vi "Read Object List.vi"(8 "error in (no error)":errorcluster, 11 "file refnum":T1) -> (0 "error out":errorcluster, 2 "Mandatory Object List":u16[](array[numeric]), 3 "Optional Object List":u16[](array[numeric]))   [LabVIEW 2013]
uses:
  <vilib>/Utility/config.llb/Config Data RefNum.ctl
  <vilib>/Utility/config.llb/NI_LVConfig.lvlib
panel:
  in  "Numeric 2":u16 format="%.0x"
  in  "Numeric":u16 format="%.0x"
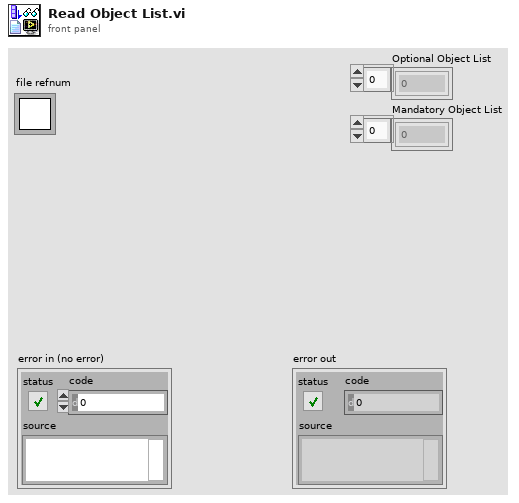
[diagram p1: front panel]
types:
  T1 = typedef "NI_LVConfig.lvlib/Config Data RefNum.ctl" = refnum<k1>
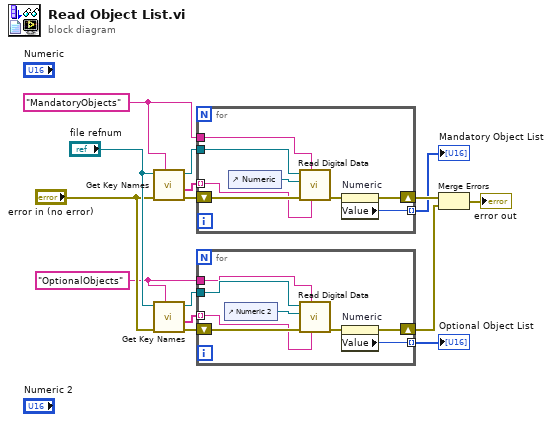
[diagram p0: block diagram]
diagram:
  w1 = "OptionalObjects"
  w13 = "MandatoryObjects"
  n1 = call <vilib>:"Get Key Names.vi"("section"=w13, "error in (no error)"="error in (no error)", "refnum"="file refnum") -> ("error out"=w14:errorcluster, "key names"=w15:string[], "refnum out"=w7:T1)  [unwired: 5 in, 1 out]
  n2 = call <vilib>:"Get Key Names.vi"("section"=w1, "error in (no error)"="error in (no error)", "refnum"="file refnum") -> ("error out"=w12:errorcluster, "key names"=w9:string[], "refnum out"=w8:T1)  [unwired: 5 in, 1 out]
  n3 = for {
    tunnel: w7 -> [w22]
    tunnel: w15 -> [w19] mode=indexing
    shift-right: [w17] -> w6
    shift-left: w14 -> [w23]
    tunnel: w13 -> [w20]
    tunnel: [w16] -> w2 mode=indexing
    n4 = control-ref of="Numeric"() -> (w21:refnum<vi>)
    n5 = call "Read Digital Data.vi"("Keyword Name"=w19, "Section Name"=w20, "error in (no error)"=w23, "DigNum Refnum"=w21, "file refnum"=w22) -> ("error out"=w18:errorcluster)  [unwired: 6 in]
    n6 = property on="Numeric" class="DigNum (strict)"(error in=w18) -> (error out=w17:errorcluster, "Value"=w16:u16)  [unwired: 1 in, 1 out]
  }
  "Mandatory Object List" <- w2
  n7 = for {
    tunnel: w8 -> [w30]
    tunnel: w9 -> [w27] mode=indexing
    shift-right: [w25] -> w5
    shift-left: w12 -> [w31]
    tunnel: w1 -> [w28]
    tunnel: [w24] -> w3 mode=indexing
    n8 = control-ref of="Numeric 2"() -> (w29:refnum<vi>)
    n9 = call "Read Digital Data.vi"("Keyword Name"=w27, "Section Name"=w28, "error in (no error)"=w31, "DigNum Refnum"=w29, "file refnum"=w30) -> ("error out"=w26:errorcluster)  [unwired: 6 in]
    n10 = property on="Numeric" class="DigNum (strict)"(error in=w26) -> (error out=w25:errorcluster, "Value"=w24:u16)  [unwired: 1 in, 1 out]
  }
  "Optional Object List" <- w3
  n11 = Merge Errors(w6, w5) -> (→"error out":errorcluster)
